vi "Get RIO and Analog Replay Strings.vi"(11 "rio/analog replay":string) -> (2 "analog replay":string, 3 "rio":string)   [LabVIEW 2015, in "Engine Simulation Toolkit System Explorer.lvlib"]
uses:
  Engine Simulation Toolkit System Explorer.lvlib
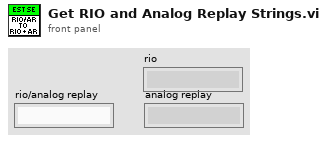
[diagram p1: front panel]
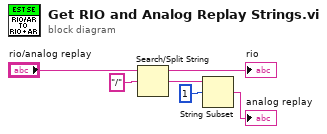
[diagram p0: block diagram]
diagram:
  n1 = Search/Split String(string="rio/analog replay", search string/char (-)="/") -> (substring before match=→"rio":string, match + rest of string=w3:string)  [unwired: 1 in, 1 out]
  n2 = String Subset(string=w3, offset (0)=1) -> (substring=→"analog replay":string)  [unwired: 1 in]
